vi "General Auto PID Simulator.vi"() -> ()   [LabVIEW 2015]
doc: "This example demonstrates how to simulate a simple control loop and a general plant model. This VI also demonstrates how you can use the PID Control VIs to autotune the PID gains."
uses:
  <vilib>/Rock Robotics/WPI/CAN/TalonSRX/WPI_CANTalonSRX_APIControlMode.ctl
  <vilib>/Rock Robotics/SystemInterfaces/AI/FPGA_AIChannel.ctl
  <vilib>/Rock Robotics/WPI/MotorControl/WPI_MotorControlOpenCANTalonSRX.vi
  <vilib>/addons/control/pid/NI_PID_autopid.lvlib
panel:
  out "Controller Output":dbl(graph)
  in  "reinitialize? (F)":bool
  in  "Autotune":bool
  in  "PID gains":T1={"proportional gain (Kc)"=20.0, "integral time (Ti, min)"=0.008, "derivative time (Td, min)"=0.001} {"derivative time (Td, min)" format="%.3f"; "integral time (Ti, min)" format="%.3f"; "proportional gain (Kc)" format="%.3f"}
  in  "Sampling Time dt (s)":dbl=0.05 min=0.001 step=0.01 format="%#.3p"
  out "Output (+/- %)":dbl(slide)=100.0 scale=-100.0..100.0
  in  "Stop":bool
  out "Process Variable and Setpoint":cluster{"initial PV":dbl, "SP(%)":dbl}(graph)
  # "Overview: This example demonstrates how to simulate a simple control loop and a general plant model.  This VI also demonstrates how you can use the PID Control VIs to autotune the PID gains.\nInstructions:\n1. Run the VI. When the PV value equals the SP value, click the Autotune button and follow the instructions in the PID Autotuning Wizard.\n2. Click Stop to stop the VI."
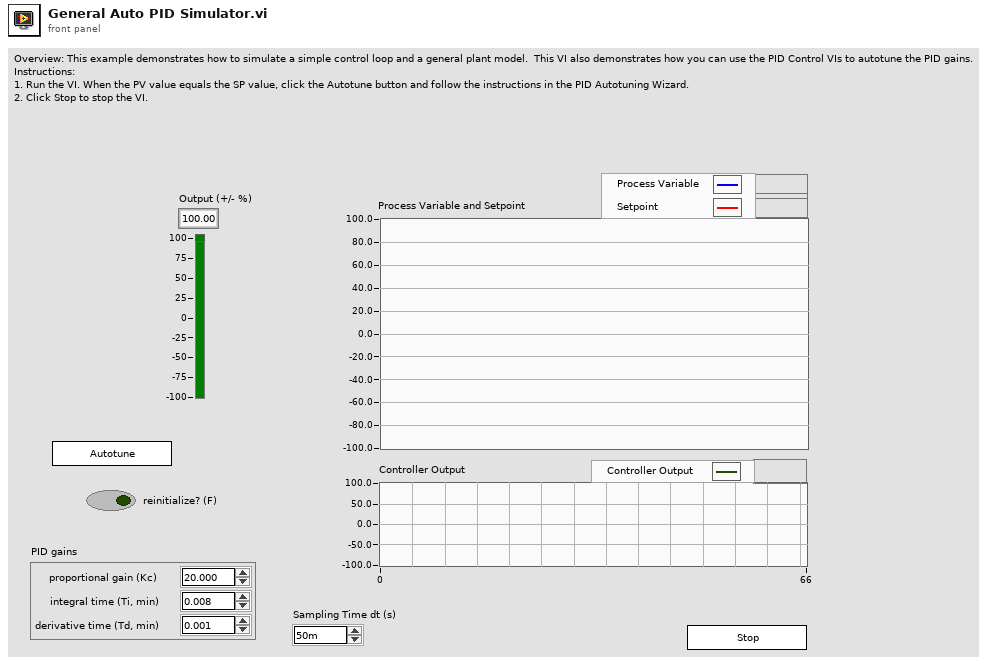
[diagram p1: front panel]
types:
  T1 = cluster{"proportional gain (Kc)":dbl, "integral time (Ti, min)":dbl, "derivative time (Td, min)":dbl}
  T2 = typedef "FPGA_AIChannel.ctl" = enum8{"AI 0", "AI 1", "AI 2", "AI 3", "AI MXP 0", "AI MXP 1", "AI MXP 2", "AI MXP 3", "Invalid"}
  T3 = typedef "WPI_CANTalonSRX_APIControlMode.ctl" = enum8{"Percent VBus", "Speed", "Position", "Slave", "Unchanged / Invalid", "Voltage Compensation", "Current", "Motion Profile"}
  T4 = typedef "WPI_PotentiometerDevRef.ctl" = cluster{"DevStatus":errorcluster, "Analog Channel":T2, "Invert Output":bool}
  T5 = typedef "WPI_MotorControlDeviceRef.ctl" = cluster{"DeviceStatus":errorcluster, "Type":T6, "PWM":cluster{"PWM Channel":T7, "DeadBand":T8}, "CAN":cluster{"Device Number":u8, "Control Mode":T9, "Semaphore":T10, "Max Vout":dbl, "TalonSRX Control Mode":T3}, "Invert":bool}
  T6 = typedef "WPI_MotorControlType.ctl" = enum16{"PWM", "CAN", "CANTalonSRX"}
  T7 = typedef "FPGA_DIOPWMChannel.ctl" = enum8{"PWM 0", "PWM 1", "PWM 2", "PWM 3", "PWM 4", "PWM 5", "PWM 6", "PWM 7", "PWM 8", "PWM 9", "PWM MXP 0", "PWM MXP 1", "PWM MXP 2", "PWM MXP 3", "PWM MXP 4", "PWM MXP 5", "PWM MXP 6", "PWM MXP 7", "PWM MXP 8", "PWM MXP 9", "Invalid"}
  T8 = typedef "WPI_PWMDeadband.ctl" = cluster{"Name":string, "maxPositivePwm":i32, "minPositivePwm":i32, "centerPwm":i32, "maxNegativePwm":i32, "minNegativePwm":i32, "angularRange":u16}
  T9 = typedef "WPI_CANJaguar_ControlMode.ctl" = enum8{"Percent VBus", "Current", "Speed", "Position", "Voltage"}
  T10 = typedef "Semaphore RefNum" = refnum<k1>
  T11 = cluster{"controller type":u16, "relay cycles":i32, "relay amplitude":dbl, "control specification":u16, "PV noise level":dbl}
  T12 = cluster{"Normalized Value":dbl, "process variable":dbl}
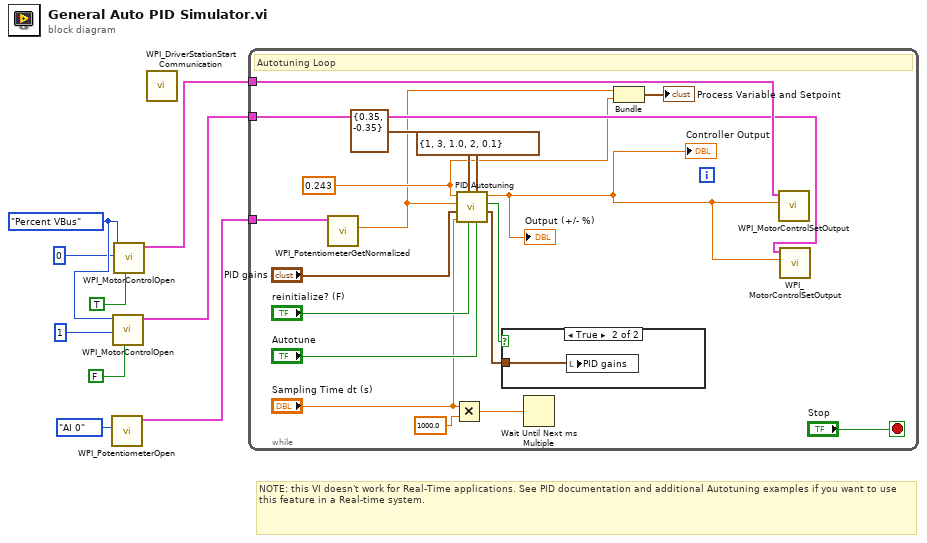
[diagram p0: block diagram]
diagram:
  w9 = WPI_CANTalonSRX_APIControlMode."Percent VBus" ("Control Mode")
  # "NOTE: this VI doesn't work for Real-Time applications. See PID documentation and additional Autotuning examples if you want to use this feature in a Real-time system."
  n1 = call <vilib>:"WPI_PotentiometerOpen.vi"("Analog Channel"=FPGA_AIChannel."AI 0") -> ("PotDevRef"=w1:T4)  [unwired: 9 in, 1 out]
  n2 = call-poly <vilib>:"WPI_MotorControlOpen.vi"("Invert"=FALSE, "Device Number"=u8 1, "Control Mode"=w9) -> ("MotorControlDeviceRef"=w3:T5)  [unwired: 7 in, 1 out]
  n3 = call-poly <vilib>:"WPI_MotorControlOpen.vi"("Invert"=TRUE, "Device Number"=u8 0, "Control Mode"=w9) -> ("MotorControlDeviceRef"=w4:T5)  [unwired: 7 in, 1 out]
  n4 = call <vilib>:"WPI_DriverStationStart Communication.vi"() -> ()  [unwired: 12 in]
  n5 = while {
    tunnel: w4 -> [w17]
    tunnel: w3 -> [w16]
    tunnel: w1 -> [w13]
    stop <- "Stop" stop-if-true
    w12 = 0.243 ("process variable")
    # "Autotuning Loop"
    n6 = call <vilib>:"WPI_PotentiometerGetNormalized.vi"("PotDevRef"=w13) -> ("Normalized Value"=w10:dbl)  [unwired: 8 in, 2 out]
    n7 = Multiply(x="Sampling Time dt (s)", y=1000.0) -> (x*y=w18:dbl)
    n8 = call <vilib>:"PID Autotuning.vi"("autotune? (F)"="Autotune", "autotuning parameters"=T11 {"controller type"=1, "relay cycles"=3, "relay amplitude"=1.0, "control specification"=2, "PV noise level"=0.1} ("autotuning initial parameters"), "reinitialize? (F)"="reinitialize? (F)", "output range"=cluster{"output high":dbl, "output low":dbl} {"output high"=0.35, "output low"=-0.35}, "dt (s)"="Sampling Time dt (s)", "PID gains"="PID gains", "process variable"=w10, "setpoint"=w12) -> ("PID gains out"=w24:T1, "tuning completed?"=w23:bool, "output"=w15:dbl)  [unwired: 1 out]
    "Output (+/- %)" <- w15
    "Controller Output" <- w15
    n9 = case shown="True" w23 {
      tunnel: w24 -> [_ w28]
      frame False {
      }
      frame True {
        n10 = local write "PID gains"(w28) -> ()
      }
    }
    n11 = Wait Until Next ms Multiple(millisecond multiple=w18) -> ()  [unwired: 1 out]
    n12 = Bundle("Normalized Value"=w10, "process variable"=w12) -> (→"Process Variable and Setpoint":T12)  [unwired: 1 in]
    n13 = call <vilib>:"WPI_MotorControlSetOutput.vi"("Output"=w15, "MotorControlDevRef"=w17) -> ()  [unwired: 7 in, 3 out]
    n14 = call <vilib>:"WPI_MotorControlSetOutput.vi"("Output"=w15, "MotorControlDevRef"=w16) -> ()  [unwired: 7 in, 3 out]
  }
